vi "iCal Get Experiment.vi"(10 "Experiment":string) -> (2 "Found":bool, 3 "Extracted Data":T1, 11 "Array":T1[](array[typedef]))   [LabVIEW 2020]
uses:
  Utilities/iCalendar/Extract iCalendar String.ctl
panel:
  in  "Path to Open":path=path "C:/Users/l121767/Downloads/calendar.ics"
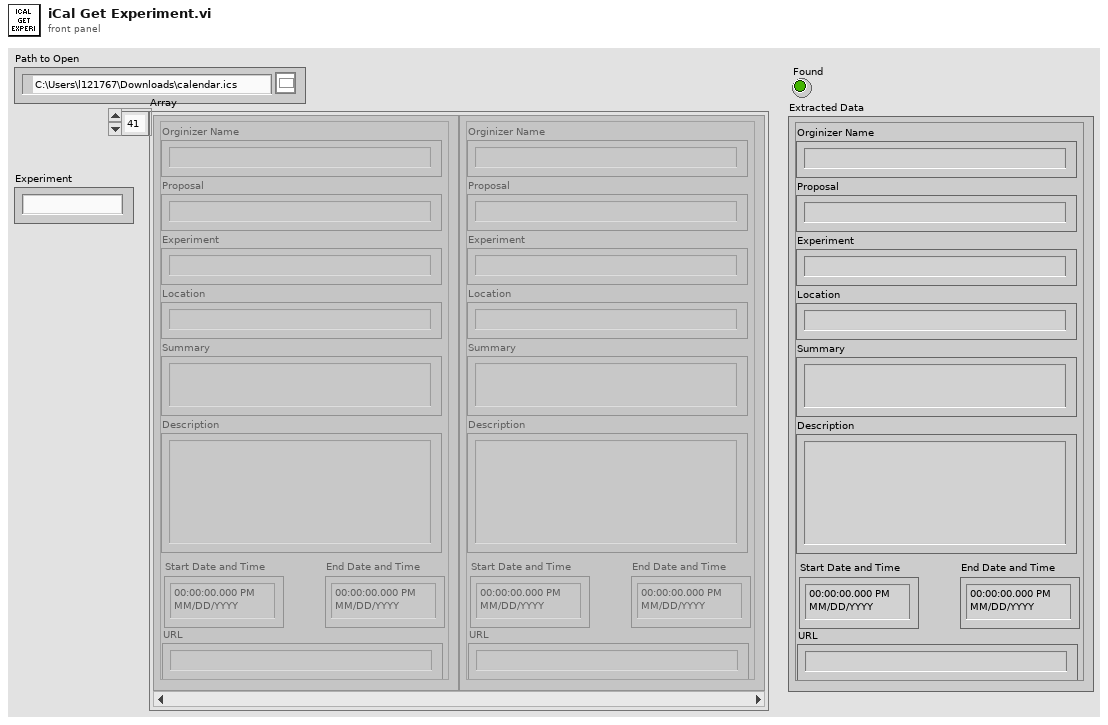
[diagram p1: front panel]
types:
  T1 = typedef "Extract iCalendar String.ctl" = cluster{"Orginizer Name":string, "Location":string, "Summary":string, "Start Date and Time":timestamp, "End Date and Time":timestamp, "Description":string, "Proposal":string, "Experiment":string, "URL":string}
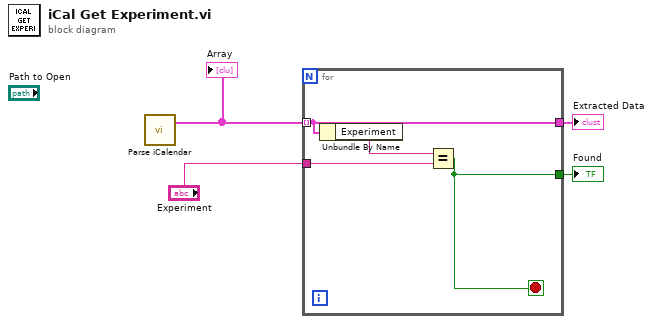
[diagram p0: block diagram]
diagram:
  n1 = call "Parse iCalendar.vi"() -> ("Events out"=w4:T1[])  [unwired: 9 in, 2 out]
  "Array" <- w4
  n2 = for {
    tunnel: w4 -> [w5] mode=indexing
    tunnel: "Experiment" -> [w7]
    tunnel: [w6] -> w2
    tunnel: [w5] -> w1
    stop <- w6 stop-if-true
    n3 = Unbundle By Name(w5) -> ("Experiment"=w8:string)
    n4 = Equal?(x=w8, y=w7) -> (x = y?=w6:bool)
  }
  "Found" <- w2
  "Extracted Data" <- w1
